vi "Clear_DAQ_Tasks.vi"(8 "error in (no error)":errorcluster, 11 "Data Cluster":T1) -> (0 "error out":errorcluster)   [LabVIEW 2017]
uses:
  Controls/ShiftRegisterCluster.ctl
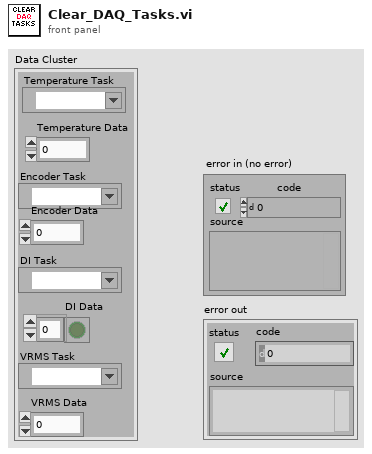
[diagram p1: front panel]
types:
  T1 = typedef "ShiftRegisterCluster.ctl" = cluster{"Temperature Task":refnum<k21>, "Temperature Data":dbl, "Encoder Task":refnum<k21>, "Encoder Data":dbl, "DI Task":refnum<k21>, "DI Data":bool[], "VRMS Task":refnum<k21>, "VRMS Data":dbl}
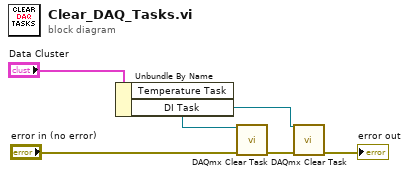
[diagram p0: block diagram]
diagram:
  n1 = Unbundle By Name("Data Cluster") -> ("Temperature Task"=w6:refnum<k21>, "DI Task"=w3:refnum<k21>)
  n2 = call <vilib>:"DAQmx Clear Task.vi"("task in"=w6, "error in"="error in (no error)") -> ("error out"=w2:errorcluster)  [unwired: 13 in]
  n3 = call <vilib>:"DAQmx Clear Task.vi"("task in"=w3, "error in"=w2) -> ("error out"=→"error out":errorcluster)  [unwired: 13 in]
